vi "Main Intermediate.vi"() -> ()   [LabVIEW 2021]
uses:
  Class Selector.ctl
  Format Key Class/Format Key Class.lvclass
  Library.lvlib
panel:
  out "Value":string
  in  "Class":T1
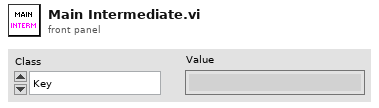
[diagram p1: front panel]
types:
  T1 = typedef "Library.lvlib/Class Selector.ctl" = enum16{"Key", "CSV"}
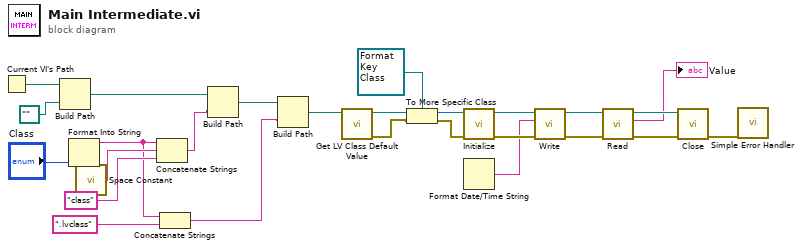
[diagram p0: block diagram]
diagram:
  n1 = Current VI's Path() -> (path=w23:path)
  n2 = Build Path(base path=w23, name or relative path=path "..") -> (appended path=w22:path)
  n3 = Format Into String("Class") -> (resulting string=w17:string)  [unwired: 3 in, 1 out]
  n4 = call <vilib>:"Space Constant.vi"() -> ("String"=w20:string)
  n5 = Concatenate Strings(w17, w20, "class" ("string")) -> (w18:string)
  n6 = Concatenate Strings(w17, ".lvclass" ("string")) -> (w15:string)
  n7 = Build Path(base path=w22, name or relative path=w18) -> (appended path=w25:path)
  n8 = Build Path(base path=w25, name or relative path=w15) -> (appended path=w24:path)
  n9 = call <vilib>:"Get LV Class Default Value.vi"("class path"=w24) -> ("error out"=w1:errorcluster, "object"=w5:refnum<class>)  [unwired: 9 in]
  n10 = To More Specific Class(target class=refnum<class "Format Key Class.lvclass"> refnum ("Library.lvlib:Format Key Class"), reference=w5, error in=w1) -> (specific class reference=w3:refnum<class "Format Key Class.lvclass">, error out=w2:errorcluster)
  n11 = call-dynamic "Initialize.vi"("error in (no error)"=w2, "Format Key Class in"=w3) -> ("error out"=w13:errorcluster, "Format Key Class out"=w14:refnum<class "Format Key Class.lvclass">)  [unwired: 8 in]
  n12 = Format Date/Time String() -> (date/time string=w7:string)  [unwired: 3 in]
  n13 = call-dynamic "Write.vi"("error in (no error)"=w13, "Value"=w7, "Format Key Class in"=w14) -> ("error out"=w11:errorcluster, "Format Key Class out"=w12:refnum<class "Format Key Class.lvclass">)  [unwired: 7 in]
  n14 = call-dynamic "Read.vi"("error in (no error)"=w11, "Format Key Class in"=w12) -> ("error out"=w9:errorcluster, "Value"=→"Value":string, "Format Key Class out"=w10:refnum<class "Format Key Class.lvclass">)  [unwired: 7 in]
  n15 = call-dynamic "Close.vi"("error in (no error)"=w9, "Format Key Class in"=w10) -> ("error out"=w8:errorcluster)  [unwired: 8 in, 1 out]
  n16 = call <vilib>:"Simple Error Handler.vi"("error in (no error)"=w8) -> ()  [unwired: 4 in, 5 out]
